vi "White_Plot.vi"() -> ()   [LabVIEW 2024]
panel:
  in  "3D?":bool=TRUE
  in  "# harmonics":i32=40
  in  "# freq":i32=48
  out "Graph":picture
  out "Linear 3":dbl[](graph)
  out "Table":string[][](table)=[["G3", "196.00", "176.02"], [" G#3/Ab3 ", "207.65", "166.14"], ["A3", "220.00", "156.82"], [" A#3/Bb3 ", "233.08", "148.02"], ["B3", "246.94", "139.71"], ["C4", "261.63", "131.87"], [" C#4/Db4 ", "277.18", "124.47"], ["D4", "293.66", "117.48"], [" D#4/Eb4 ", "311.13", "110.89"], ["E4", "329.63", "104.66"], ["F4", "349.23", "98.79"], [" F#4/Gb4 ", "369.99", "93.24"], ["G4", "392.00", "88.01"], [" G#4/Ab4 ", "415.30", "83.07"], ["A4", "440.00", "78.41"], [" A#4/Bb4 ", "466.16", "74.01"], ["B4", "493.88", "69.85"], ["C5", "523.25", "65.93"], [" C#5/Db5 ", "554.37", "62.23"], ["D5", "587.33", "58.74"], [" D#5/Eb5 ", "622.25", "55.44"], ["E5", "659.25", "52.33"], ["F5", "698.46", "49.39"], [" F#5/Gb5 ", "739.99", "46.62"], ["G5", "783.99", "44.01"], [" G#5/Ab5 ", "830.61", "41.54"], ["A5", "880.00", "39.20"], [" A#5/Bb5 ", "932.33", "37.00"], ["B5", "987.77", "34.93"], ["C6", "1046.50", "32.97"], [" C#6/Db6 ", "1108.73", "31.12"], ["D6", "1174.66", "29.37"], [" D#6/Eb6 ", "1244.51", "27.72"], ["E6", "1318.51", "26.17"], ["F6", "1396.91", "24.70"], [" F#6/Gb6 ", "1479.98", "23.31"], ["G6", "1567.98", "22.00"], [" G#6/Ab6 ", "1661.22", "20.77"], ["A6", "1760.00", "19.60"], [" A#6/Bb6 ", "1864.66", "18.50"], ["B6", "1975.53", "17.46"], ["C7", "2093.00", "16.48"], [" C#7/Db7 ", "2217.46", "15.56"], ["D7", "2349.32", "14.69"], [" D#7/Eb7 ", "2489.02", "13.86"], ["E7", "2637.02", "13.08"], ["F7", "2793.83", "12.35"], [" F#7/Gb7 ", "2959.96", "11.66"], ["G7", "3135.96", "11.00"], [" G#7/Ab7 ", "3322.44", "10.38"], ["A7", "3520.00", "9.80"], ["A#7/Bb7 ", "3729.31", "9.25"], ["B7", "3951.07", "8.73"]]
  out "White Plot":dbl[][](graph)=[[-15.822857410944914, 7.169908015047404, 16.453602515846452, 9.79965030999062, 12.997590613201496, 7.879466749616089, 10.093922203026008, 9.503590939660562, 8.623723226558473, 16.60785785860815, 14.404444279162526, 14.413714318535067, 12.801392593344564, 13.247072776605792, 10.01640688894864, 11.922856715797167, 11.579669448522216, 9.774767477968338, 13.50409882639825, 11.125877771744337, 12.036086120580674, 11.679993562515316, 9.422467767327603, 8.74241616397563, 11.86609961234582, 8.837250159996685, 9.761825934571196, 7.763187815648874, 9.020410987177032, 7.014374865580616, 7.771723147846208, 9.149402493790028, 8.711203714066933, 7.300943007093607, 6.475876910582946, 5.687649840054397, 4.294857191976305, 2.9824739109932263, 3.558447863833478, 3.8571915688284752, 3.1301445178639513, 2.2135406593674762, 2.6646928913204175, 5.370179221724156, 5.098998307683456, 3.442823577997187, 4.310150857466436, 2.5777668361267727, 2.1281801953591226, 4.364374146914016, 4.628769773490856, 3.050932446619056, 1.8049940967710707, 2.9953965256379074, 4.024621763870566, 3.3954107627976753, 3.3044912589221997, 2.4186779875283455, 2.2829954685473024, 1.5267660826453944, 3.580693082165283, 4.691396887602427, 4.496812075475368, 1.8653537803452915, 1.4013554377729536, 3.6906066961530195, 4.442268726051577, 3.999058597017191, 3.8038705097351238, 4.397915080691513, 5.722214349179877, 5.335627877417151, 4.835367390217918, 4.209441156541385], [-12.180068359471946, 9.47271638143391, 11.861949484232062, 7.425865492399204, 12.256026417684204, 9.817051660246758, 10.486751171116548, 8.521420531462221, 11.084719464204351, 11.843996722777344, 11.402862141396728, 15.23631209325063, 13.392135899956624, 9.68420636474486, 11.041721726842987, 12.069482899381756, 9.758982739591723, 13.601182648506903, 12.330785827221575, 11.160911134531336, 11.356879880726362, 7.924019588452684, 10.134176477118944, 9.337960611342137, 8.09103987055938, 9.22021713273934, 8.07936042516819, 7.783677762366652, 7.670825679478881, 8.58451322242002, 9.20459639558007, 7.601654164606488, 6.589583578423768, 5.63269972579298, 4.098916462823988, 2.816911409099338, 3.0202404062141683, 3.9319209714259706, 2.7221182053703896, 2.287040356766285, 3.426017473887808, 5.8169908251903815, 4.607702711576101, 4.431916726309753, 2.4475777152883893, 2.390023811991205, 4.0391433919584205, 4.497258314509233, 3.1416195861988223, 1.8940067081074106, 2.9919941647817887, 4.144967821131656, 3.4983477291297755, 3.0766237410916237, 2.4616288221473335, 2.025879696650072, 2.390342410719292, 4.277287448334607, 4.587884448574216, 3.4778429301162896, 0.7089295713816293, 3.0760930869177554, 4.473679460407606, 4.0591828394555485, 3.8705860116815316, 4.229043575463752, 5.72614495051614, 5.319402040956591, 4.737315445081279, 4.409058180544939, 7.319357628493833, 7.511184942650122, nan, nan], [-5.885477455411069, 22.747309895103335, 8.571026934955228, 10.631146404555924, 12.481311976967252, 2.554225465854174, 9.57281078906281, 8.906772304360073, 16.004162100598027, 12.462973659331551, 15.891471252984548, 11.593668018519391, 7.569504777659003, 10.645541256171501, 13.154801975082313, 9.940246596811285, 13.601030348629644, 12.587067797976026, 11.386493827271591, 11.908101271256983, 7.488851157221038, 10.64988344303355, 8.729981788618032, 9.67617830219448, 7.430399295809881, 9.325897207879262, 7.713495622640119, 7.937058426043473, 9.412336481296235, 8.44041826124095, 6.81137025681428, 5.741206551485999, 4.196771570009812, 2.8176610124870605, 2.9004629708875513, 4.097579608707368, 2.1072273528903946, 2.14020060678187, 4.653272305817894, 5.286049612132836, 3.3784803553775085, 3.702126258436116, 2.7654960400919064, 2.9053502186454097, 4.442142853753732, 3.7551145881774923, 2.618877061787681, 3.0448210595721066, 4.024621763870566, 3.478359537119439, 3.0305558907297483, 2.4514128934898647, 1.7659460681341412, 3.001189548741205, 4.5494206732501885, 4.5439959972432415, 1.93132217445224, 1.5710448269044186, 4.214991416857855, 4.205909617451128, 3.688209902015211, 3.9048563022111527, 5.6695885527357825, 5.344602036373121, 4.86434821005183, 4.286388075590183, 7.28519203579175, 7.468931380585905, nan, nan, nan, nan, nan, nan], [-0.06679092623095685, 5.9512028385521285, 10.550677320865308, 9.930527994578824, 6.993345713448309, 13.19934940121479, 6.842631039933865, 10.851508223577568, 13.628633729491398, 13.486001469456848, 12.392346702650665, 12.329462765321475, 9.906078882792585, 13.185500800964627, 10.527796238055, 13.538059972664065, 12.631621829754607, 11.56557238538305, 12.178621838373765, 8.160113794727984, 11.807326174560227, 8.315256490740271, 9.995443106447725, 7.926574683762661, 7.5209094520459, 7.595761333377005, 9.258956235100353, 8.709253441332823, 6.912974306112546, 5.7900751405823145, 4.426640566206553, 2.8995845784718006, 2.9404271404808178, 4.1132409978606, 2.016978828641223, 2.3273211035240307, 5.370179221724156, 4.727834303520317, 3.4960186437594003, 2.4834667780577115, 2.370674237513908, 4.309775388323441, 4.6275620102501165, 3.4326073291453003, 2.3292804320951794, 3.5426939244790856, 3.4607481659710104, 3.205588709002087, 2.4616288221473335, 1.8237846834675677, 3.07762744374316, 4.639293671130645, 4.484150891841475, 1.2867114137621893, 2.229029510358182, 4.546816107809168, 4.0627887464089945, 3.820397563184051, 4.827515564609741, 5.603490686973788, 5.047229515490782, 4.262666949455136, 6.6448947128913884, 7.547945791198859, nan, nan, nan, nan, nan, nan, nan, nan, nan, nan], [-9.344667816257722, 4.244669313078728, 13.486125316915409, 13.094378121232179, 10.934985499191942, 10.969394424902926, 8.149875351149982, 16.17196406942285, 12.307125679025798, 15.838955217854185, 13.68776808239587, 9.086402993347855, 11.89535518469069, 11.309299082627167, 13.16086636832803, 12.421260531230828, 11.564444079903872, 12.194137840334278, 8.629539268985829, 11.521919403384475, 7.9705542389989965, 8.635077142839865, 8.98348507654315, 7.533120314391358, 7.933349008039486, 9.353130890147217, 7.260391198183328, 6.00282059965275, 4.882044458627183, 3.329854429875671, 3.4351959125082625, 3.981915562634895, 2.0422470210716943, 2.363540775262209, 5.554775356500078, 4.620974147082772, 4.431916726309753, 2.4158009423493976, 2.2450694538507037, 4.382888764296612, 3.690878547303072, 2.100273235109203, 3.1005170842276675, 4.030068741417608, 3.5794688066416747, 2.4104240443830833, 2.204879186889591, 2.654281588741468, 4.5494206732501885, 4.497291320824779, 1.16026801395088, 2.57603869143784, 4.464469750191363, 3.98722049530139, 3.7273878959093394, 5.51115933066042, 5.345607016793251, 4.7592681316140535, 4.756096630552154, 7.962402663276343, nan, nan, nan, nan, nan, nan, nan, nan, nan, nan, nan, nan, nan, nan], [4.495120162184895, 13.985362155289769, 9.377295739540564, 12.625497153155338, 0.8387429892509517, 9.483697833085, 11.342112398098969, 13.168578617924844, 14.48005500511427, 11.766417762398191, 8.773116067094456, 11.990276006519434, 10.630088386397178, 11.745159148404174, 11.277923992872136, 11.495510054684, 12.173338214703639, 8.753430719726211, 9.94377887592828, 9.035366727359964, 7.60771415168687, 9.151498324410488, 7.716567610576571, 9.197411461472111, 8.72945471632181, 6.827932720227885, 5.5782398022007715, 3.818629867369304, 3.801802075008843, 3.862641268790388, 2.542055580947122, 2.219495798826627, 5.477875809679944, 4.607289890110012, 4.6001678886823925, 2.632168960569751, 2.9170156818658617, 4.518727656417259, 3.018384636239385, 2.0689048333787934, 3.60312130385135, 3.4103198047098977, 2.73460526052433, 2.3996537614839495, 1.7078389388496584, 4.214020979715472, 4.58203557182271, 1.6982817337953633, 2.229029510358182, 4.473679460407606, 3.971695541146179, 3.8238402433274383, 5.691590757456483, 5.304270428621472, 4.49171410852563, 6.055643116558502, 7.548932056964128, nan, nan, nan, nan, nan, nan, nan, nan, nan, nan, nan, nan, nan, nan, nan, nan, nan], [13.097779924858958, 11.892653292360205, 7.425865492399204, 11.995483103694378, 12.209946181141515, 8.632502427674618, 16.03361146220543, 12.012490491959868, 15.167469112067542, 12.801026640500856, 10.319686516510362, 11.854002172700419, 10.569365974893152, 10.814881735395765, 11.146189365713397, 12.194248148495019, 8.748125507681426, 9.158974932094678, 9.643726287555944, 6.839141487811177, 7.62262211096071, 7.978471838110728, 9.409345757811728, 7.4719941908799115, 5.89508696110647, 4.549559238379041, 2.8329262240308166, 3.5512358786678493, 3.0826713678365723, 2.1798800503699685, 4.8738232773801045, 4.643107230678488, 4.5285774048855245, 2.663728303437794, 3.236532437037895, 4.524009831593173, 3.4326073291453003, 2.895744804885218, 4.184066546975382, 3.5340657158672037, 2.41578167283685, 1.9329133805441994, 3.455478743884907, 4.646303921847641, 3.216310242555467, 1.4846492373541254, 4.535268814052143, 4.041784997714145, 3.7273878959093394, 5.662698335731556, 5.279210482898922, 4.369648917005725, 6.732002300386507, 7.408346263474273, nan, nan, nan, nan, nan, nan, nan, nan, nan, nan, nan, nan, nan, nan, nan, nan, nan, nan, nan, nan], [7.895064263226152, 16.152081103706976, 10.948750887051569, 7.4084152389650235, 9.317199204226888, 8.705209597074596, 11.322025923707702, 14.341946150830157, 11.598981069706829, 10.047953078457896, 12.700931876505683, 9.86849718139139, 13.4192107587786, 12.226204330445649, 12.022984199251553, 8.710968660048405, 9.01492683298541, 9.698567989150428, 7.634071360950655, 7.057631773313469, 7.923916987074666, 8.797429392782725, 6.90833426317093, 5.731548474079624, 3.728749911510101, 3.6323672048390017, 4.1204519965516235, 2.158244650911513, 3.463154295704249, 5.227247777143099, 3.778756542885264, 2.503570165746064, 3.0700806819127164, 4.564966161048909, 3.448075220817637, 3.004160147016636, 4.030068741417608, 3.4012259354462366, 2.4958555184726836, 1.394183780899068, 4.254163884664907, 4.51310831573678, 0.8281665461571968, 3.5513755723540874, 4.19763147514362, 3.857034004134162, 5.359141924045354, 5.331334267315509, 4.494659298047918, 6.611579230959828, 7.330328105202425, nan, nan, nan, nan, nan, nan, nan, nan, nan, nan, nan, nan, nan, nan, nan, nan, nan, nan, nan, nan, nan, nan, nan], [5.808712966015297, 11.962858494244827, 9.869350196028638, 9.935126100100902, 9.955583374475342, 10.919461733597506, 13.502616083645275, 15.290723093324146, 12.20346765671218, 10.859114803457963, 11.14684467998269, 13.580332821380717, 12.483817890016418, 11.280730621925859, 8.316469145652944, 9.619487616435206, 9.735043082678711, 7.99757234526729, 7.3252251549429275, 8.487859247014995, 8.69527001142367, 6.667220964453577, 4.872264577388724, 2.8334466628451875, 3.733073455114439, 2.8151441597529474, 2.387278451138525, 5.832308495890199, 3.342487828876453, 2.4704752542187776, 2.431740933369616, 4.492156099398968, 3.4936793559801793, 2.998809116413649, 3.8862884155838175, 3.140425933099566, 2.3996537614839495, 2.166519044232647, 4.694704649952228, 3.731875855634196, 1.5420462692537376, 4.516210413111985, 3.8593770001007597, 4.09594686056774, 5.552568652455308, 4.8160469468028015, 5.534211676046848, 7.539130252494122, nan, nan, nan, nan, nan, nan, nan, nan, nan, nan, nan, nan, nan, nan, nan, nan, nan, nan, nan, nan, nan, nan, nan, nan, nan, nan], [5.762229988947823, 8.625061351427034, 12.816600388842986, 2.3142081977501108, 7.964220149799971, 16.08232762025348, 11.934643485354222, 11.680003073529404, 8.94575667467797, 13.235193921552309, 10.817252264783967, 12.49573894209741, 11.59507492097173, 7.50031277717608, 11.27824009580914, 9.658541014291105, 8.038693745674086, 7.636146636143229, 9.059043112750032, 8.568695400787043, 5.935235851047387, 4.294857191976305, 3.768793811522621, 4.022580401787657, 2.23607994569368, 4.432231482037543, 4.597081720844399, 3.9089653690552155, 2.3502793010782375, 4.422290103951007, 3.089067016677462, 3.0194261803891873, 3.957616184659349, 3.108697373871045, 2.3264776710754838, 2.8533378076967493, 4.648860863126981, 2.2143677735245233, 2.8358806732543624, 4.2402978947643355, 3.829748301086648, 5.606807341636645, 5.154247222961745, 4.211482835734502, 7.997990183260382, nan, nan, nan, nan, nan, nan, nan, nan, nan, nan, nan, nan, nan, nan, nan, nan, nan, nan, nan, nan, nan, nan, nan, nan, nan, nan, nan, nan, nan], [2.528266008474195, 10.556653813477347, 12.586673750177113, 13.17094145926411, 9.834382466472526, 13.36717214222206, 16.53354972397999, 12.429477667859734, 12.016465201016828, 10.62132542077988, 12.27604321807317, 11.546782890383799, 8.010925601510856, 11.671349220302558, 9.157293349074113, 7.851461957529721, 7.683843536695038, 9.251144623099112, 7.79689340825985, 5.843450840679828, 3.7897398670238305, 3.0202404062141683, 3.1833672624708003, 2.2799998036034075, 5.759019800590238, 3.2686160141829768, 2.693193287927012, 4.253368350269509, 3.637787555511764, 2.1915345565809057, 4.1729800527958405, 3.283189659207614, 2.3618578824912544, 2.944115738585389, 4.629738165403333, 1.5000455743043992, 3.5513755723540874, 4.08563195053453, 3.8967397830623645, 5.637934409142621, 4.78171719733308, 6.362564282821344, nan, nan, nan, nan, nan, nan, nan, nan, nan, nan, nan, nan, nan, nan, nan, nan, nan, nan, nan, nan, nan, nan, nan, nan, nan, nan, nan, nan, nan, nan, nan, nan], [10.417740899297241, 13.529642908648395, 11.97067061328179, 10.854476984485506, 10.808063963524017, 12.150230842564941, 11.610307715448103, 9.296625779128128, 11.656068128799276, 13.0251732675396, 12.867895189310497, 12.197160361122704, 10.465395615707017, 7.879861779463652, 6.838089673426325, 7.446645731589564, 9.255352199392712, 7.3559816801421, 5.73383671890083, 3.3434142339764628, 3.6436711984058268, 2.1072273528903946, 3.3806724784560958, 4.6165264833310165, 3.503797026806772, 2.1604551771331546, 4.596486798870554, 2.3190310199499216, 3.6366338741671034, 3.573767970967409, 2.5208315137591235, 2.4435560644335093, 4.6481876844465795, 1.3941701429186892, 3.8610368961054102, 4.006251356063548, 4.09594686056774, 5.393925636662418, 4.3287273879143635, 7.854594230124476, nan, nan, nan, nan, nan, nan, nan, nan, nan, nan, nan, nan, nan, nan, nan, nan, nan, nan, nan, nan, nan, nan, nan, nan, nan, nan, nan, nan, nan, nan, nan, nan, nan, nan], [7.169908015047404, 9.79965030999062, 7.879466749616089, 9.503590939660562, 16.60785785860815, 14.413714318535067, 13.247072776605792, 11.922856715797167, 9.774767477968338, 11.125877771744337, 11.679993562515316, 8.74241616397563, 8.837250159996685, 7.763187815648874, 7.014374865580616, 9.149402493790028, 7.300943007093607, 5.687649840054397, 2.9824739109932263, 3.8571915688284752, 2.2135406593674762, 5.370179221724156, 3.442823577997187, 2.5777668361267727, 4.364374146914016, 3.050932446619056, 2.9953965256379074, 3.3954107627976753, 2.4186779875283455, 1.5267660826453944, 4.691396887602427, 1.8653537803452915, 3.6906066961530195, 3.999058597017191, 4.397915080691513, 5.335627877417151, 4.209441156541385, 7.571009971852272, nan, nan, nan, nan, nan, nan, nan, nan, nan, nan, nan, nan, nan, nan, nan, nan, nan, nan, nan, nan, nan, nan, nan, nan, nan, nan, nan, nan, nan, nan, nan, nan, nan, nan, nan, nan], [9.47271638143391, 7.425865492399204, 9.817051660246758, 8.521420531462221, 11.843996722777344, 15.23631209325063, 9.68420636474486, 12.069482899381756, 13.601182648506903, 11.160911134531336, 7.924019588452684, 9.337960611342137, 9.22021713273934, 7.783677762366652, 8.58451322242002, 7.601654164606488, 5.63269972579298, 2.816911409099338, 3.9319209714259706, 2.287040356766285, 5.8169908251903815, 4.431916726309753, 2.390023811991205, 4.497258314509233, 1.8940067081074106, 4.144967821131656, 3.0766237410916237, 2.025879696650072, 4.277287448334607, 3.4778429301162896, 3.0760930869177554, 4.0591828394555485, 4.229043575463752, 5.319402040956591, 4.409058180544939, 7.511184942650122, nan, nan, nan, nan, nan, nan, nan, nan, nan, nan, nan, nan, nan, nan, nan, nan, nan, nan, nan, nan, nan, nan, nan, nan, nan, nan, nan, nan, nan, nan, nan, nan, nan, nan, nan, nan, nan, nan], [22.747309895103335, 10.631146404555924, 2.554225465854174, 8.906772304360073, 12.462973659331551, 11.593668018519391, 10.645541256171501, 9.940246596811285, 12.587067797976026, 11.908101271256983, 10.64988344303355, 9.67617830219448, 9.325897207879262, 7.937058426043473, 8.44041826124095, 5.741206551485999, 2.8176610124870605, 4.097579608707368, 2.14020060678187, 5.286049612132836, 3.702126258436116, 2.9053502186454097, 3.7551145881774923, 3.0448210595721066, 3.478359537119439, 2.4514128934898647, 3.001189548741205, 4.5439959972432415, 1.5710448269044186, 4.205909617451128, 3.9048563022111527, 5.344602036373121, 4.286388075590183, 7.468931380585905, nan, nan, nan, nan, nan, nan, nan, nan, nan, nan, nan, nan, nan, nan, nan, nan, nan, nan, nan, nan, nan, nan, nan, nan, nan, nan, nan, nan, nan, nan, nan, nan, nan, nan, nan, nan, nan, nan, nan, nan], [5.9512028385521285, 9.930527994578824, 13.19934940121479, 10.851508223577568, 13.486001469456848, 12.329462765321475, 13.185500800964627, 13.538059972664065, 11.56557238538305, 8.160113794727984, 8.315256490740271, 7.926574683762661, 7.595761333377005, 8.709253441332823, 5.7900751405823145, 2.8995845784718006, 4.1132409978606, 2.3273211035240307, 4.727834303520317, 2.4834667780577115, 4.309775388323441, 3.4326073291453003, 3.5426939244790856, 3.205588709002087, 1.8237846834675677, 4.639293671130645, 1.2867114137621893, 4.546816107809168, 3.820397563184051, 5.603490686973788, 4.262666949455136, 7.547945791198859, nan, nan, nan, nan, nan, nan, nan, nan, nan, nan, nan, nan, nan, nan, nan, nan, nan, nan, nan, nan, nan, nan, nan, nan, nan, nan, nan, nan, nan, nan, nan, nan, nan, nan, nan, nan, nan, nan, nan, nan, nan, nan], [4.244669313078728, 13.094378121232179, 10.969394424902926, 16.17196406942285, 15.838955217854185, 9.086402993347855, 11.309299082627167, 12.421260531230828, 12.194137840334278, 11.521919403384475, 8.635077142839865, 7.533120314391358, 9.353130890147217, 6.00282059965275, 3.329854429875671, 3.981915562634895, 2.363540775262209, 4.620974147082772, 2.4158009423493976, 4.382888764296612, 2.100273235109203, 4.030068741417608, 2.4104240443830833, 2.654281588741468, 4.497291320824779, 2.57603869143784, 3.98722049530139, 5.51115933066042, 4.7592681316140535, 7.962402663276343, nan, nan, nan, nan, nan, nan, nan, nan, nan, nan, nan, nan, nan, nan, nan, nan, nan, nan, nan, nan, nan, nan, nan, nan, nan, nan, nan, nan, nan, nan, nan, nan, nan, nan, nan, nan, nan, nan, nan, nan, nan, nan, nan, nan], [13.985362155289769, 12.625497153155338, 9.483697833085, 13.168578617924844, 11.766417762398191, 11.999722965033303, 11.745159148404174, 11.495510054684, 8.753430719726211, 9.035366727359964, 9.151498324410488, 9.197411461472111, 6.828168806409786, 3.818629867369304, 3.862641268790388, 2.219495798826627, 4.607289890110012, 2.628043128908101, 4.518727656417259, 2.0689048333787934, 3.4103198047098977, 2.3996537614839495, 4.212878835986508, 1.6982817337953633, 4.475582270539688, 3.8238402433274383, 5.304270428621472, 6.041086368054112, nan, nan, nan, nan, nan, nan, nan, nan, nan, nan, nan, nan, nan, nan, nan, nan, nan, nan, nan, nan, nan, nan, nan, nan, nan, nan, nan, nan, nan, nan, nan, nan, nan, nan, nan, nan, nan, nan, nan, nan, nan, nan, nan, nan, nan, nan], [11.892653292360205, 11.995483103694378, 8.632502427674618, 12.012490491959868, 12.801026640500856, 11.854002172700419, 10.814881735395765, 12.194248148495019, 9.158974932094678, 6.839141487811177, 7.978471838110728, 7.4719941908799115, 4.549559238379041, 3.5592785731800918, 2.1798800503699685, 4.643107230678488, 2.663728303437794, 4.524009831593173, 2.895744804885218, 3.5340657158672037, 1.9329133805441994, 4.648860863126981, 1.497309647101138, 4.039557123837463, 5.662698335731556, 4.369648917005725, 7.408346263474273, nan, nan, nan, nan, nan, nan, nan, nan, nan, nan, nan, nan, nan, nan, nan, nan, nan, nan, nan, nan, nan, nan, nan, nan, nan, nan, nan, nan, nan, nan, nan, nan, nan, nan, nan, nan, nan, nan, nan, nan, nan, nan, nan, nan, nan, nan, nan], [16.152081103706976, 7.4084152389650235, 8.705209597074596, 14.341946150830157, 10.063797037599498, 9.86849718139139, 12.226204330445649, 8.710968660048405, 9.698567989150428, 7.057631773313469, 8.797429392782725, 5.731548474079624, 3.6323672048390017, 2.16607898518815, 5.215414187271073, 2.503570165746064, 4.564966161048909, 3.004160147016636, 3.4012259354462366, 1.394183780899068, 4.51310831573678, 3.5513755723540874, 3.8520537496426552, 5.331311886490694, 6.633836575860997, nan, nan, nan, nan, nan, nan, nan, nan, nan, nan, nan, nan, nan, nan, nan, nan, nan, nan, nan, nan, nan, nan, nan, nan, nan, nan, nan, nan, nan, nan, nan, nan, nan, nan, nan, nan, nan, nan, nan, nan, nan, nan, nan, nan, nan, nan, nan, nan, nan], [11.962858494244827, 9.935126100100902, 10.919461733597506, 15.290723093324146, 10.859114803457963, 13.572484108763845, 11.280730621925859, 9.619487616435206, 7.99757234526729, 8.487859247014995, 6.685052356637073, 2.8334466628451875, 2.8151441597529474, 5.832308495890199, 2.4704752542187776, 4.492156099398968, 2.998809116413649, 3.1435035089529744, 2.166519044232647, 3.731875855634196, 4.516210413111985, 4.09594686056774, 4.819247249097264, 7.539130252494122, nan, nan, nan, nan, nan, nan, nan, nan, nan, nan, nan, nan, nan, nan, nan, nan, nan, nan, nan, nan, nan, nan, nan, nan, nan, nan, nan, nan, nan, nan, nan, nan, nan, nan, nan, nan, nan, nan, nan, nan, nan, nan, nan, nan, nan, nan, nan, nan, nan, nan], [8.625061351427034, 2.3142081977501108, 16.08232762025348, 11.680003073529404, 13.271706146053102, 12.49573894209741, 7.50031277717608, 9.658541014291105, 7.636146636143229, 8.568695400787043, 4.294857191976305, 4.022580401787657, 4.432231482037543, 3.925349436259578, 4.417662656808038, 3.0194261803891873, 3.108697373871045, 2.8533378076967493, 2.2143677735245233, 4.2402978947643355, 5.606807341636645, 4.211482835734502, nan, nan, nan, nan, nan, nan, nan, nan, nan, nan, nan, nan, nan, nan, nan, nan, nan, nan, nan, nan, nan, nan, nan, nan, nan, nan, nan, nan, nan, nan, nan, nan, nan, nan, nan, nan, nan, nan, nan, nan, nan, nan, nan, nan, nan, nan, nan, nan, nan, nan, nan, nan], [10.556653813477347, 13.17094145926411, 13.36717214222206, 12.429477667859734, 10.62132542077988, 11.546782890383799, 11.671349220302558, 7.851461957529721, 9.251144623099112, 5.843450840679828, 3.0202404062141683, 2.2799998036034075, 3.2686160141829768, 4.253368350269509, 2.1915345565809057, 3.283189659207614, 2.944115738585389, 1.5000455743043992, 4.08563195053453, 5.637934409142621, 6.362564282821344, nan, nan, nan, nan, nan, nan, nan, nan, nan, nan, nan, nan, nan, nan, nan, nan, nan, nan, nan, nan, nan, nan, nan, nan, nan, nan, nan, nan, nan, nan, nan, nan, nan, nan, nan, nan, nan, nan, nan, nan, nan, nan, nan, nan, nan, nan, nan, nan, nan, nan, nan, nan, nan], [13.529642908648395, 10.854476984485506, 12.150230842564941, 9.296625779128128, 13.0251732675396, 12.197160361122704, 7.879861779463652, 7.446645731589564, 7.3559816801421, 3.3434142339764628, 2.1072273528903946, 4.6165264833310165, 2.1604551771331546, 2.2922134193623487, 3.573767970967409, 2.4435560644335093, 1.3850708807733045, 4.006251356063548, 5.393925636662418, 7.858609077314341, nan, nan, nan, nan, nan, nan, nan, nan, nan, nan, nan, nan, nan, nan, nan, nan, nan, nan, nan, nan, nan, nan, nan, nan, nan, nan, nan, nan, nan, nan, nan, nan, nan, nan, nan, nan, nan, nan, nan, nan, nan, nan, nan, nan, nan, nan, nan, nan, nan, nan, nan, nan, nan, nan], [9.79965030999062, 9.503590939660562, 14.413714318535067, 11.922856715797167, 11.125877771744337, 8.736728380321734, 7.763187815648874, 9.149402493790028, 5.687649840054397, 3.8571915688284752, 5.36100117488154, 2.5777668361267727, 3.050932446619056, 3.3954107627976753, 1.5267660826453944, 1.8653537803452915, 3.999058597017191, 5.3362858699787985, 7.571009971852272, nan, nan, nan, nan, nan, nan, nan, nan, nan, nan, nan, nan, nan, nan, nan, nan, nan, nan, nan, nan, nan, nan, nan, nan, nan, nan, nan, nan, nan, nan, nan, nan, nan, nan, nan, nan, nan, nan, nan, nan, nan, nan, nan, nan, nan, nan, nan, nan, nan, nan, nan, nan, nan, nan, nan], [7.425865492399204, 8.521420531462221, 15.23631209325063, 12.069482899381756, 11.160911134531336, 9.337960611342137, 7.783677762366652, 7.601654164606488, 2.817502156808565, 2.278956579158044, 4.431916726309753, 4.497258314509233, 4.144967821131656, 2.025879696650072, 3.4778429301162896, 4.0591828394555485, 5.319402040956591, 7.511184942650122, nan, nan, nan, nan, nan, nan, nan, nan, nan, nan, nan, nan, nan, nan, nan, nan, nan, nan, nan, nan, nan, nan, nan, nan, nan, nan, nan, nan, nan, nan, nan, nan, nan, nan, nan, nan, nan, nan, nan, nan, nan, nan, nan, nan, nan, nan, nan, nan, nan, nan, nan, nan, nan, nan, nan, nan], [10.631146404555924, 8.906772304360073, 11.593668018519391, 9.940246596811285, 11.908101271256983, 9.67617830219448, 7.937058426043473, 5.741206551485999, 4.097579608707368, 5.286049612132836, 2.9053502186454097, 3.0448210595721066, 2.4514128934898647, 4.5439959972432415, 4.205909617451128, 5.344602036373121, 7.468931380585905, nan, nan, nan, nan, nan, nan, nan, nan, nan, nan, nan, nan, nan, nan, nan, nan, nan, nan, nan, nan, nan, nan, nan, nan, nan, nan, nan, nan, nan, nan, nan, nan, nan, nan, nan, nan, nan, nan, nan, nan, nan, nan, nan, nan, nan, nan, nan, nan, nan, nan, nan, nan, nan, nan, nan, nan, nan], [9.930527994578824, 10.851508223577568, 12.329462765321475, 13.538059972664065, 8.160113794727984, 7.926574683762661, 8.708197096116653, 2.897045588666481, 2.3273211035240307, 2.4834667780577115, 3.4326073291453003, 3.205588709002087, 4.639293671130645, 4.546816107809168, 5.603490686973788, 7.547945791198859, nan, nan, nan, nan, nan, nan, nan, nan, nan, nan, nan, nan, nan, nan, nan, nan, nan, nan, nan, nan, nan, nan, nan, nan, nan, nan, nan, nan, nan, nan, nan, nan, nan, nan, nan, nan, nan, nan, nan, nan, nan, nan, nan, nan, nan, nan, nan, nan, nan, nan, nan, nan, nan, nan, nan, nan, nan, nan], [13.094378121232179, 16.17196406942285, 9.086402993347855, 12.429928748343853, 11.521919403384475, 7.533120314391358, 6.00282059965275, 3.981915562634895, 4.620974147082772, 4.382888764296612, 4.030068741417608, 2.654281588741468, 2.57603869143784, 5.51115933066042, 7.962402663276343, nan, nan, nan, nan, nan, nan, nan, nan, nan, nan, nan, nan, nan, nan, nan, nan, nan, nan, nan, nan, nan, nan, nan, nan, nan, nan, nan, nan, nan, nan, nan, nan, nan, nan, nan, nan, nan, nan, nan, nan, nan, nan, nan, nan, nan, nan, nan, nan, nan, nan, nan, nan, nan, nan, nan, nan, nan, nan, nan], [12.625497153155338, 13.168578617924844, 11.999722965033303, 11.495510054684, 9.035366727359964, 9.197411461472111, 3.818629867369304, 2.219495798826627, 2.628043128908101, 2.0689048333787934, 2.3996537614839495, 1.6982817337953633, 3.8238402433274383, 6.041086368054112, nan, nan, nan, nan, nan, nan, nan, nan, nan, nan, nan, nan, nan, nan, nan, nan, nan, nan, nan, nan, nan, nan, nan, nan, nan, nan, nan, nan, nan, nan, nan, nan, nan, nan, nan, nan, nan, nan, nan, nan, nan, nan, nan, nan, nan, nan, nan, nan, nan, nan, nan, nan, nan, nan, nan, nan, nan, nan, nan, nan], [11.995483103694378, 12.012490491959868, 11.854002172700419, 12.194248148495019, 6.839141487811177, 7.4719941908799115, 3.5592785731800918, 4.643107230678488, 4.524009831593173, 3.5340657158672037, 4.648860863126981, 4.041784997714145, 4.369648917005725, nan, nan, nan, nan, nan, nan, nan, nan, nan, nan, nan, nan, nan, nan, nan, nan, nan, nan, nan, nan, nan, nan, nan, nan, nan, nan, nan, nan, nan, nan, nan, nan, nan, nan, nan, nan, nan, nan, nan, nan, nan, nan, nan, nan, nan, nan, nan, nan, nan, nan, nan, nan, nan, nan, nan, nan, nan, nan, nan, nan, nan], [7.4084152389650235, 14.341946150830157, 9.86849718139139, 8.710968660048405, 7.057631773313469, 5.731548474079624, 2.16607898518815, 2.503570165746064, 3.004160147016636, 1.394183780899068, 3.5513755723540874, 5.331311886490694, nan, nan, nan, nan, nan, nan, nan, nan, nan, nan, nan, nan, nan, nan, nan, nan, nan, nan, nan, nan, nan, nan, nan, nan, nan, nan, nan, nan, nan, nan, nan, nan, nan, nan, nan, nan, nan, nan, nan, nan, nan, nan, nan, nan, nan, nan, nan, nan, nan, nan, nan, nan, nan, nan, nan, nan, nan, nan, nan, nan, nan, nan], [9.935126100100902, 15.290723093324146, 13.580332821380717, 9.619487616435206, 8.487859247014995, 2.8334466628451875, 5.832308495890199, 4.492156099398968, 3.140425933099566, 3.731875855634196, 4.09594686056774, 7.539130252494122, nan, nan, nan, nan, nan, nan, nan, nan, nan, nan, nan, nan, nan, nan, nan, nan, nan, nan, nan, nan, nan, nan, nan, nan, nan, nan, nan, nan, nan, nan, nan, nan, nan, nan, nan, nan, nan, nan, nan, nan, nan, nan, nan, nan, nan, nan, nan, nan, nan, nan, nan, nan, nan, nan, nan, nan, nan, nan, nan, nan, nan, nan], [2.3142081977501108, 11.680003073529404, 12.49573894209741, 9.658541014291105, 8.568695400787043, 4.022580401787657, 3.925349436259578, 3.0194261803891873, 2.8533378076967493, 4.2402978947643355, 4.211482835734502, nan, nan, nan, nan, nan, nan, nan, nan, nan, nan, nan, nan, nan, nan, nan, nan, nan, nan, nan, nan, nan, nan, nan, nan, nan, nan, nan, nan, nan, nan, nan, nan, nan, nan, nan, nan, nan, nan, nan, nan, nan, nan, nan, nan, nan, nan, nan, nan, nan, nan, nan, nan, nan, nan, nan, nan, nan, nan, nan, nan, nan, nan, nan], [13.17094145926411, 12.430599773585541, 11.546782890383799, 7.851461957529721, 5.843450840679828, 2.2763753001640605, 4.253368350269509, 3.283189659207614, 1.5000455743043992, 5.642117518487332, nan, nan, nan, nan, nan, nan, nan, nan, nan, nan, nan, nan, nan, nan, nan, nan, nan, nan, nan, nan, nan, nan, nan, nan, nan, nan, nan, nan, nan, nan, nan, nan, nan, nan, nan, nan, nan, nan, nan, nan, nan, nan, nan, nan, nan, nan, nan, nan, nan, nan, nan, nan, nan, nan, nan, nan, nan, nan, nan, nan, nan, nan, nan, nan], [10.854476984485506, 9.296625779128128, 12.197160361122704, 7.446645731589564, 3.3434142339764628, 4.6165264833310165, 2.2922134193623487, 2.4435560644335093, 4.006251356063548, 7.858609077314341, nan, nan, nan, nan, nan, nan, nan, nan, nan, nan, nan, nan, nan, nan, nan, nan, nan, nan, nan, nan, nan, nan, nan, nan, nan, nan, nan, nan, nan, nan, nan, nan, nan, nan, nan, nan, nan, nan, nan, nan, nan, nan, nan, nan, nan, nan, nan, nan, nan, nan, nan, nan, nan, nan, nan, nan, nan, nan, nan, nan, nan, nan, nan, nan], [9.503590939660562, 11.922856715797167, 8.736728380321734, 9.149402493790028, 3.8571915688284752, 2.5777668361267727, 3.3954107627976753, 1.8653537803452915, 5.3362858699787985, nan, nan, nan, nan, nan, nan, nan, nan, nan, nan, nan, nan, nan, nan, nan, nan, nan, nan, nan, nan, nan, nan, nan, nan, nan, nan, nan, nan, nan, nan, nan, nan, nan, nan, nan, nan, nan, nan, nan, nan, nan, nan, nan, nan, nan, nan, nan, nan, nan, nan, nan, nan, nan, nan, nan, nan, nan, nan, nan, nan, nan, nan, nan, nan, nan], [8.521420531462221, 12.069482899381756, 9.337960611342137, 7.601654164606488, 2.278956579158044, 4.497258314509233, 2.025879696650072, 4.0591828394555485, 7.511184942650122, nan, nan, nan, nan, nan, nan, nan, nan, nan, nan, nan, nan, nan, nan, nan, nan, nan, nan, nan, nan, nan, nan, nan, nan, nan, nan, nan, nan, nan, nan, nan, nan, nan, nan, nan, nan, nan, nan, nan, nan, nan, nan, nan, nan, nan, nan, nan, nan, nan, nan, nan, nan, nan, nan, nan, nan, nan, nan, nan, nan, nan, nan, nan, nan, nan], [8.906772304360073, 9.940246596811285, 9.67617830219448, 5.741206551485999, 5.286049612132836, 3.0448210595721066, 4.5439959972432415, 5.344602036373121, nan, nan, nan, nan, nan, nan, nan, nan, nan, nan, nan, nan, nan, nan, nan, nan, nan, nan, nan, nan, nan, nan, nan, nan, nan, nan, nan, nan, nan, nan, nan, nan, nan, nan, nan, nan, nan, nan, nan, nan, nan, nan, nan, nan, nan, nan, nan, nan, nan, nan, nan, nan, nan, nan, nan, nan, nan, nan, nan, nan, nan, nan, nan, nan, nan, nan], [10.851508223577568, 13.538059972664065, 7.926574683762661, 2.897045588666481, 2.4834667780577115, 3.205588709002087, 4.546816107809168, 7.547945791198859, nan, nan, nan, nan, nan, nan, nan, nan, nan, nan, nan, nan, nan, nan, nan, nan, nan, nan, nan, nan, nan, nan, nan, nan, nan, nan, nan, nan, nan, nan, nan, nan, nan, nan, nan, nan, nan, nan, nan, nan, nan, nan, nan, nan, nan, nan, nan, nan, nan, nan, nan, nan, nan, nan, nan, nan, nan, nan, nan, nan, nan, nan, nan, nan, nan, nan], [16.17196406942285, 12.429928748343853, 7.533120314391358, 3.981915562634895, 4.382888764296612, 2.654281588741468, 5.51115933066042, nan, nan, nan, nan, nan, nan, nan, nan, nan, nan, nan, nan, nan, nan, nan, nan, nan, nan, nan, nan, nan, nan, nan, nan, nan, nan, nan, nan, nan, nan, nan, nan, nan, nan, nan, nan, nan, nan, nan, nan, nan, nan, nan, nan, nan, nan, nan, nan, nan, nan, nan, nan, nan, nan, nan, nan, nan, nan, nan, nan, nan, nan, nan, nan, nan, nan, nan], [13.168578617924844, 11.495510054684, 9.197411461472111, 2.219495798826627, 2.0689048333787934, 1.6982817337953633, 6.041086368054112, nan, nan, nan, nan, nan, nan, nan, nan, nan, nan, nan, nan, nan, nan, nan, nan, nan, nan, nan, nan, nan, nan, nan, nan, nan, nan, nan, nan, nan, nan, nan, nan, nan, nan, nan, nan, nan, nan, nan, nan, nan, nan, nan, nan, nan, nan, nan, nan, nan, nan, nan, nan, nan, nan, nan, nan, nan, nan, nan, nan, nan, nan, nan, nan, nan, nan, nan], [12.012490491959868, 12.194248148495019, 7.4719941908799115, 4.643107230678488, 3.5340657158672037, 4.041784997714145, nan, nan, nan, nan, nan, nan, nan, nan, nan, nan, nan, nan, nan, nan, nan, nan, nan, nan, nan, nan, nan, nan, nan, nan, nan, nan, nan, nan, nan, nan, nan, nan, nan, nan, nan, nan, nan, nan, nan, nan, nan, nan, nan, nan, nan, nan, nan, nan, nan, nan, nan, nan, nan, nan, nan, nan, nan, nan, nan, nan, nan, nan, nan, nan, nan, nan, nan, nan], [14.341946150830157, 8.710968660048405, 5.731548474079624, 2.503570165746064, 1.394183780899068, 5.331311886490694, nan, nan, nan, nan, nan, nan, nan, nan, nan, nan, nan, nan, nan, nan, nan, nan, nan, nan, nan, nan, nan, nan, nan, nan, nan, nan, nan, nan, nan, nan, nan, nan, nan, nan, nan, nan, nan, nan, nan, nan, nan, nan, nan, nan, nan, nan, nan, nan, nan, nan, nan, nan, nan, nan, nan, nan, nan, nan, nan, nan, nan, nan, nan, nan, nan, nan, nan, nan], [15.290723093324146, 9.619487616435206, 2.8334466628451875, 4.492156099398968, 3.731875855634196, 7.539130252494122, nan, nan, nan, nan, nan, nan, nan, nan, nan, nan, nan, nan, nan, nan, nan, nan, nan, nan, nan, nan, nan, nan, nan, nan, nan, nan, nan, nan, nan, nan, nan, nan, nan, nan, nan, nan, nan, nan, nan, nan, nan, nan, nan, nan, nan, nan, nan, nan, nan, nan, nan, nan, nan, nan, nan, nan, nan, nan, nan, nan, nan, nan, nan, nan, nan, nan, nan, nan], [11.680003073529404, 9.658541014291105, 4.022580401787657, 3.0194261803891873, 4.2402978947643355, nan, nan, nan, nan, nan, nan, nan, nan, nan, nan, nan, nan, nan, nan, nan, nan, nan, nan, nan, nan, nan, nan, nan, nan, nan, nan, nan, nan, nan, nan, nan, nan, nan, nan, nan, nan, nan, nan, nan, nan, nan, nan, nan, nan, nan, nan, nan, nan, nan, nan, nan, nan, nan, nan, nan, nan, nan, nan, nan, nan, nan, nan, nan, nan, nan, nan, nan, nan, nan], [12.429477667859734, 7.851461957529721, 2.2799998036034075, 3.283189659207614, 5.637934409142621, nan, nan, nan, nan, nan, nan, nan, nan, nan, nan, nan, nan, nan, nan, nan, nan, nan, nan, nan, nan, nan, nan, nan, nan, nan, nan, nan, nan, nan, nan, nan, nan, nan, nan, nan, nan, nan, nan, nan, nan, nan, nan, nan, nan, nan, nan, nan, nan, nan, nan, nan, nan, nan, nan, nan, nan, nan, nan, nan, nan, nan, nan, nan, nan, nan, nan, nan, nan, nan], [9.296625779128128, 7.446645731589564, 4.6165264833310165, 2.4435560644335093, 7.858609077314341, nan, nan, nan, nan, nan, nan, nan, nan, nan, nan, nan, nan, nan, nan, nan, nan, nan, nan, nan, nan, nan, nan, nan, nan, nan, nan, nan, nan, nan, nan, nan, nan, nan, nan, nan, nan, nan, nan, nan, nan, nan, nan, nan, nan, nan, nan, nan, nan, nan, nan, nan, nan, nan, nan, nan, nan, nan, nan, nan, nan, nan, nan, nan, nan, nan, nan, nan, nan, nan], [11.922856715797167, 9.149402493790028, 2.5777668361267727, 1.8653537803452915, nan, nan, nan, nan, nan, nan, nan, nan, nan, nan, nan, nan, nan, nan, nan, nan, nan, nan, nan, nan, nan, nan, nan, nan, nan, nan, nan, nan, nan, nan, nan, nan, nan, nan, nan, nan, nan, nan, nan, nan, nan, nan, nan, nan, nan, nan, nan, nan, nan, nan, nan, nan, nan, nan, nan, nan, nan, nan, nan, nan, nan, nan, nan, nan, nan, nan, nan, nan, nan, nan], [12.069482899381756, 7.601654164606488, 4.497258314509233, 4.0591828394555485, nan, nan, nan, nan, nan, nan, nan, nan, nan, nan, nan, nan, nan, nan, nan, nan, nan, nan, nan, nan, nan, nan, nan, nan, nan, nan, nan, nan, nan, nan, nan, nan, nan, nan, nan, nan, nan, nan, nan, nan, nan, nan, nan, nan, nan, nan, nan, nan, nan, nan, nan, nan, nan, nan, nan, nan, nan, nan, nan, nan, nan, nan, nan, nan, nan, nan, nan, nan, nan, nan], [9.940246596811285, 5.741206551485999, 3.0448210595721066, 5.344602036373121, nan, nan, nan, nan, nan, nan, nan, nan, nan, nan, nan, nan, nan, nan, nan, nan, nan, nan, nan, nan, nan, nan, nan, nan, nan, nan, nan, nan, nan, nan, nan, nan, nan, nan, nan, nan, nan, nan, nan, nan, nan, nan, nan, nan, nan, nan, nan, nan, nan, nan, nan, nan, nan, nan, nan, nan, nan, nan, nan, nan, nan, nan, nan, nan, nan, nan, nan, nan, nan, nan], [13.538059972664065, 2.897045588666481, 3.205588709002087, 7.547945791198859, nan, nan, nan, nan, nan, nan, nan, nan, nan, nan, nan, nan, nan, nan, nan, nan, nan, nan, nan, nan, nan, nan, nan, nan, nan, nan, nan, nan, nan, nan, nan, nan, nan, nan, nan, nan, nan, nan, nan, nan, nan, nan, nan, nan, nan, nan, nan, nan, nan, nan, nan, nan, nan, nan, nan, nan, nan, nan, nan, nan, nan, nan, nan, nan, nan, nan, nan, nan, nan, nan], [12.429928748343853, 3.981915562634895, 2.654281588741468, nan, nan, nan, nan, nan, nan, nan, nan, nan, nan, nan, nan, nan, nan, nan, nan, nan, nan, nan, nan, nan, nan, nan, nan, nan, nan, nan, nan, nan, nan, nan, nan, nan, nan, nan, nan, nan, nan, nan, nan, nan, nan, nan, nan, nan, nan, nan, nan, nan, nan, nan, nan, nan, nan, nan, nan, nan, nan, nan, nan, nan, nan, nan, nan, nan, nan, nan, nan, nan, nan, nan]]
  in  "path":path=path "/Users/crogers/Documents/Personal/Violin Stuff/GS Huberman Rad with chinrest/Averages/GS_Huberman_21 with ch rst H.AvR"
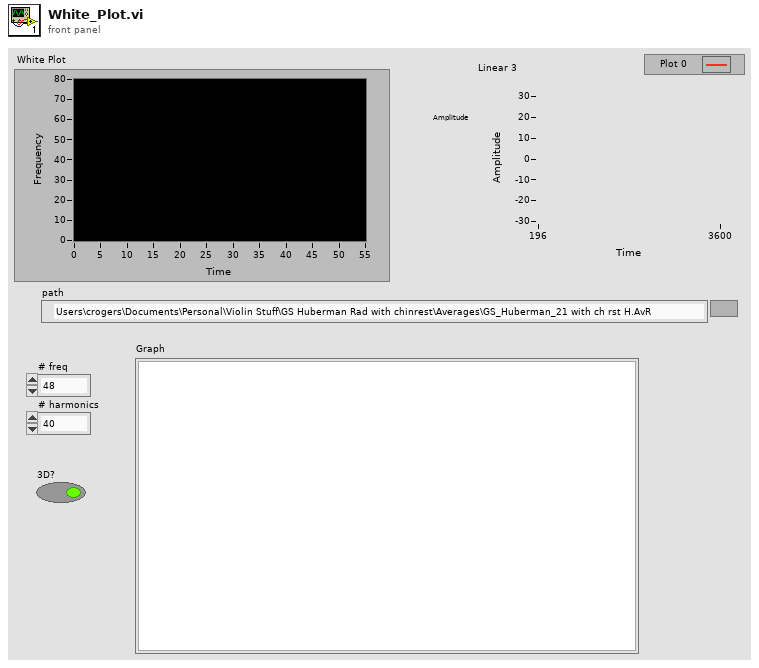
[diagram p1: front panel]
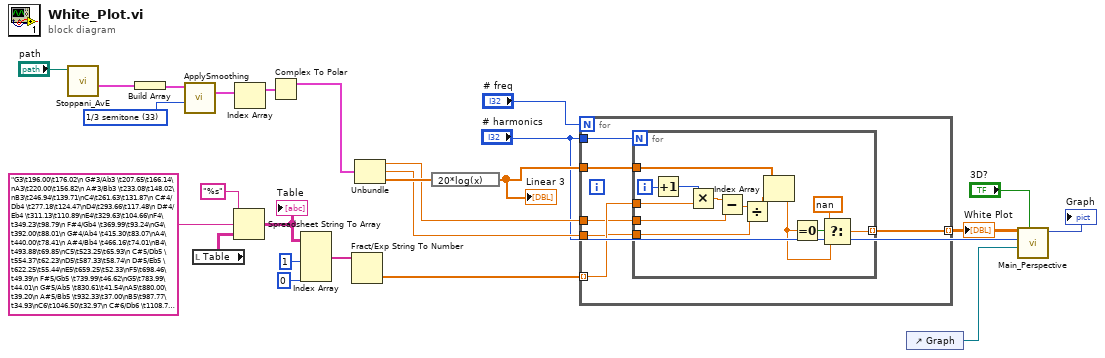
[diagram p0: block diagram]
diagram:
  w8 = u16 33 items=["No smoothing"=0, "1/4 semitone"=25, "1/3 semitone"=33, "1/2 semitone"=50, "1 semitone"=100, "2 semitones"=200] ("Smoothing")
  n1 = call "Stoppani_AvE.vi"("file (use dialog)"="path") -> ("Complex FRF"=w15:cluster{"t0":dbl, "df":dbl, "Y":cdb[]})  [unwired: 7 in, 3 out]
  n2 = Build Array(w15) -> (w18:cluster{"t0":dbl, "df":dbl, "Y":cdb[]}[])
  n3 = call "ApplySmoothing.vi"("Smoothing"=w8, "Complex FRF"=w18) -> ("Complex FRF Out"=w17:cluster{dbl, "df":dbl, cdb[]}[])  [unwired: 9 in]
  n4 = local read "Table"() -> (w23:string[][])
  n5 = Spreadsheet String To Array(format string="%s", spreadsheet string="G3\t196.00\t176.02\n G#3/Ab3 \t207.65\t166.14\nA3\t220.00\t156.82\n A#3/Bb3 \t233.08\t148.02\nB3\t246.94\t139.71\nC4\t261.63\t131.87\n C#4/Db4 \t277.18\t124.47\nD4\t293.66\t117.48\n D#4/Eb4 \t311.13\t110.89\nE4\t329.63\t104.66\nF4\t349.23\t98.79\n F#4/Gb4 \t369.99\t93.24\nG4\t392.00\t88.01\n G#4/Ab4 \t415.30\t83.07\nA4\t440.00\t78.41\n A#4/Bb4 \t466.16\t74.01\nB4\t493.88\t69.85\nC5\t523.25\t65.93\n C#5/Db5 \t554.37\t62.23\nD5\t587.33\t58.74\n D#5/Eb5 \t622.25\t55.44\nE5\t659.25\t52.33\nF5\t698.46\t49.39\n F#5/Gb5 \t739.99\t46.62\nG5\t783.99\t44.01\n G#5/Ab5 \t830.61\t41.54\nA5\t880.00\t39.20\n A#5/Bb5 \t932.33\t37.00\nB5\t987.77\t34.93\nC6\t1046.50\t32.97\n C#6/Db6 \t1108.73\t31.12\nD6\t1174.66\t29.37\n D#6/Eb6 \t1244.51\t27.72\nE6\t1318.51\t26.17\nF6\t1396.91\t24.70\n F#6/Gb6 \t1479.98\t23.31\nG6\t1567.98\t22.00\n G#6/Ab6 \t1661.22\t20.77\nA6\t1760.00\t19.60\n A#6/Bb6 \t1864.66\t18.50\nB6\t1975.53\t17.46\nC7\t2093.00\t16.48\n C#7/Db7 \t2217.46\t15.56\nD7\t2349.32\t14.69\n D#7/Eb7 \t2489.02\t13.86\nE7\t2637.02\t13.08\nF7\t2793.83\t12.35\n F#7/Gb7 \t2959.96\t11.66\nG7\t3135.96\t11.00\n G#7/Ab7 \t3322.44\t10.38\nA7\t3520.00\t9.80\nA#7/Bb7 \t3729.31\t9.25\nB7\t3951.07\t8.73\nC8\t4186.01\t8.24\n C#8/Db8 \t4434.92\t7.78\nD8\t4698.63\t7.34\n D#8/Eb8 \t4978.03\t6.93\nE8\t5274.04\t6.54\nF8\t5587.65\t6.17\n F#8/Gb8 \t5919.91\t5.83\nG8\t6271.93\t5.50\n G#8/Ab8 \t6644.88\t5.19\nA8\t7040.00\t4.90\n A#8/Bb8 \t7458.62\t4.63\nB8\t7902.13\t4.37" ("Notes"), array type (2D Dbl)=w23) -> (array=w22:string[][])  [unwired: 1 in]
  "Table" <- w22
  n6 = Index Array(array=w17) -> (element=w16:cluster{dbl, "df":dbl, cdb[]})  [unwired: 1 in]
  n7 = Complex To Polar(r * e^(i*theta)=w16) -> (r=w14:cluster{dbl, "df":dbl, dbl[]})  [unwired: 1 out]
  n8 = Index Array(array=w22, index (col) #1=1 ("disabled index (col)"), index (col) #2=0 ("disabled index (col)")) -> (element #1=w20:string[])  [unwired: 2 in, 1 out]
  n9 = Fract/Exp String To Number(string=w20) -> (number=w19:dbl[])  [unwired: 3 in, 1 out]
  n10 = Unbundle(w14) -> (w11:dbl, "df"=w10:dbl, w13:dbl[])
  n11 = expression code="20*log(x)"(w13) -> (w12:dbl[])
  "Linear 3" <- w12
  n12 = for {
    N: "# freq" -> [_]
    tunnel: w12 -> [w31]
    tunnel: [w27] -> w6 mode=indexing
    tunnel: w19 -> [w30] mode=indexing
    tunnel: w11 -> [w28]
    tunnel: w10 -> [w29]
    tunnel: "# harmonics" -> [w26]
    n13 = for {
      N: w26 -> [_]
      tunnel: w31 -> [w44]
      tunnel: w30 -> [w41]
      tunnel: w28 -> [w40]
      tunnel: w29 -> [w39]
      tunnel: [w37] -> w27 mode=indexing
      i -> [w32]
      n14 = Increment(x=w32) -> (x+1=w33:i32)
      n15 = Multiply(x=w33, y=w41) -> (x*y=w43:dbl)
      n16 = Subtract(x=w43, y=w40) -> (x-y=w42:dbl)
      n17 = Divide(x=w42, y=w39) -> (x/y=w35:dbl)
      n18 = Index Array(array=w44, index=w35) -> (element=w34:dbl)
      n19 = Equal To 0?(x=w34) -> (x = 0?=w38:bool)
      n20 = Select(t=nan, s=w38, f=w34) -> (s? t:f=w37:dbl)
    }
  }
  "White Plot" <- w6
  n21 = control-ref of="Graph"() -> (w4:refnum<vi>)
  n22 = call "Main_Perspective.vi"("3D?"="3D?", "labels"=w4, "White Plot"="# harmonics", "picture in"=w6) -> ("Graph"=→"Graph":picture)  [unwired: 7 in]
